vi "start_stimulation.vi"(8 "error in (no error)":errorcluster, 11 "DL090503StimulatorScaffold in":refnum<class "StimulatorDL090503.lvclass">) -> (0 "error out":errorcluster, 3 "DL090503StimulatorScaffold out":refnum<class "StimulatorDL090503.lvclass">)   [LabVIEW 2010, in "StimulatorDL090503.lvclass"]
uses:
  StimulatorDL090503.lvclass
  StimulatorDL090503.lvclass/StimulatorDL090503.ctl
  SignalWriter/GenericSignalWriter/GenericSignalWriter/GenericSignalWriter.lvclass
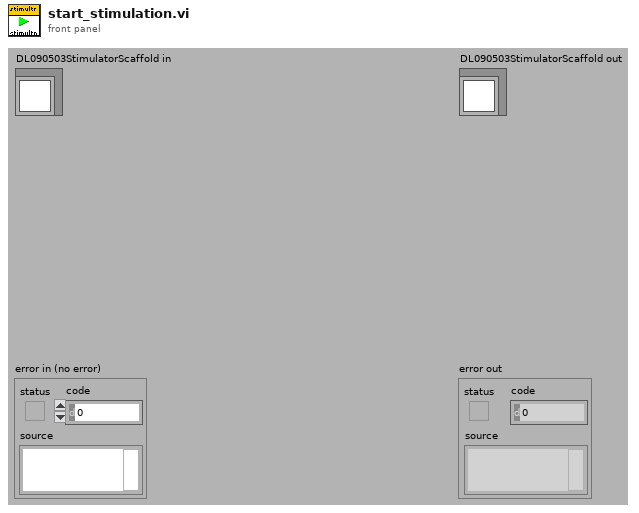
[diagram p1: front panel]
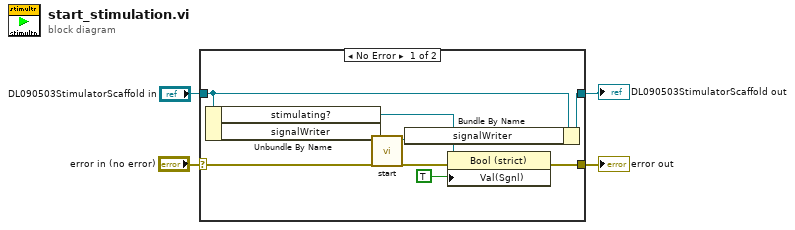
[diagram p0: block diagram]
diagram:
  n1 = case shown="No Error" "error in (no error)" {
    selector: "error in (no error)" -> [w10 w15]
    tunnel: [w12 w15] -> w4
    tunnel: [w5 w14] -> w3
    tunnel: "DL090503StimulatorScaffold in" -> [w6 w14]
    frame No Error {
      n2 = Unbundle By Name(w6) -> ("stimulating?"=w13:refnum<vi>, "signalWriter"=w8:refnum<class "GenericSignalWriter.lvclass">)
      n3 = call-dynamic "start.vi"("error in (no error)"=w10, "WriteSignalsGenericPlugin in"=w8) -> ("error out"=w9:errorcluster, "WriteSignalsGenericPlugin out"=w7:refnum<class "GenericSignalWriter.lvclass">)  [unwired: 8 out]
      n4 = Bundle By Name(cluster=w6, "signalWriter"=w7) -> (w5:refnum<class "StimulatorDL090503.lvclass">)
      n5 = property class="Bool (strict)"(reference=w13, error in=w9, "Val(Sgnl)"=TRUE ("Value (Signaling)")) -> (error out=w12:errorcluster)  [unwired: 1 out]
    }
    frame Error {
    }
  }
  "error out" <- w4
  "DL090503StimulatorScaffold out" <- w3
